vi "BLM status.vi"(2 "error in (no error)":errorcluster, 4 "Motor Address":string="0", 5 "Porty Address":refnum<visa-resource-name>) -> (0 "error out":errorcluster, 1 "Motor is moving":bool)   [LabVIEW 2019]
uses:
  BLM_IgnoreAlarms.vi
panel:
  out "BLM Status":bool[](array[boolean])
  out "Response":string
  # "SC command - Response Details:\nHex Value Status Code bit definition\n0001 Motor Enabled (Motor Disabled if this bit = 0)\n0002 Sampling (for Quick Tuner)\n0004 Drive Fault (check Alarm Code)\n0008 In Position (motor is in position)\n0010 Moving (motor is moving)\n0020 Jogging (currently in jog mode)\n0040 Stopping (in the process of stopping from a stop command)\n0080 Waiting (for an input)\n0100 Saving (parameter data is being saved)\n0200 Alarm present (check Alarm Code)\n0400 Homing (executing an SH command)\n0800 Wait Time (executing a WT command)\n1000 Wizard running (Timing Wizard is running)\n2000 Checking encoder (Timing Wizard is running)\n4000 Q Program is running\n8000 Initializing (happens at power up)"
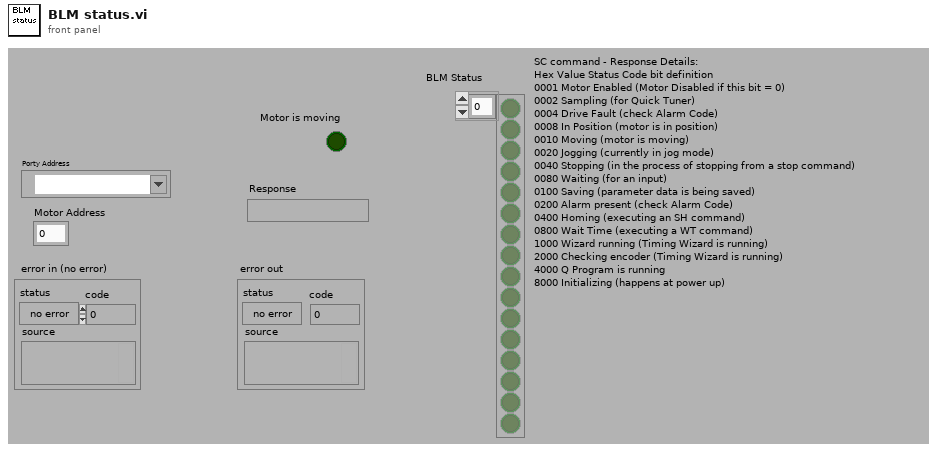
[diagram p1: front panel]
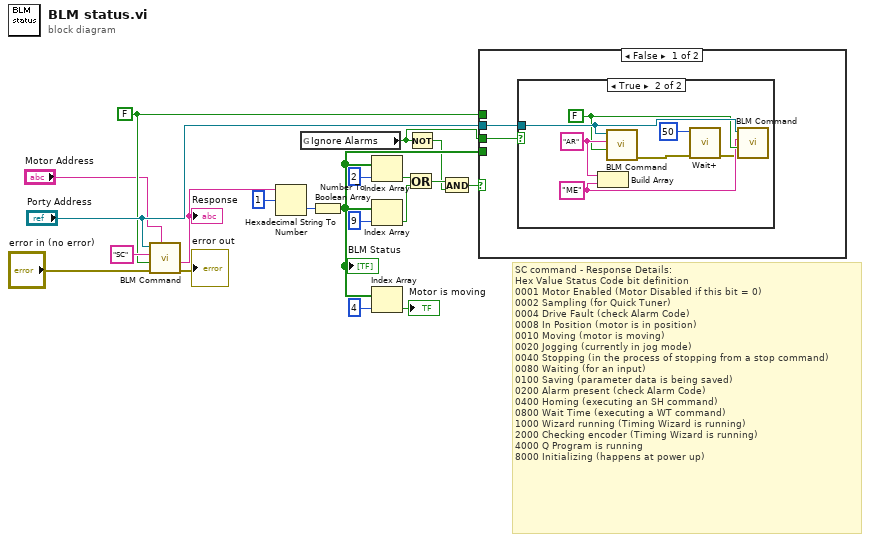
[diagram p0: block diagram]
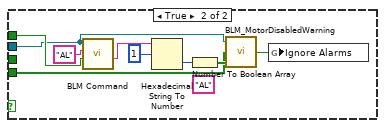
[diagram p3: hidden frame]
diagram:
  w6 = FALSE
  # "SC command - Response Details:\nHex Value Status Code bit definition\n0001 Motor Enabled (Motor Disabled if this bit = 0)\n0002 Sampling (for Quick Tuner)\n0004 Drive Fault (check Alarm Code)\n0008 In Position (motor is in position)\n0010 Moving (motor is moving)\n0020 Jogging (currently in jog mode)\n0040 Stopping (in the process of stopping from a stop command)\n0080 Waiting (for an input)\n0100 Saving (parameter data is being saved)\n0200 Alarm present (check Alarm Code)\n0400 Homing (executing an SH command)\n0800 Wait Time (executing a WT command)\n1000 Wizard running (Timing Wizard is running)\n2000 Checking encoder (Timing Wizard is running)\n4000 Q Program is running\n8000 Initializing (happens at power up)"
  n1 = call "BLM Command.vi"("Motor Address"="Motor Address", "error in (no error)"="error in (no error)", "Read Echo?"=w6, "Command"="SC", "Port Address"="Porty Address") -> ("error out"=→"error out":errorcluster, "Response"=w17:string)  [unwired: 1 in, 3 out]
  "Response" <- w17
  n2 = Hexadecimal String To Number(string=w17, offset=u32 1 ("initial scan location")) -> (number=w15:u32)  [unwired: 1 in, 1 out]
  n3 = global read "BLM_IgnoreAlarms.vi" "Ignore Alarms"() -> (w2:bool)
  n4 = Number To Boolean Array(number=w15) -> (Boolean array=w8:bool[])
  "BLM Status" <- w8
  n5 = Index Array(array=w8, index=2) -> (element=w12:bool)
  n6 = Index Array(array=w8, index=9) -> (element=w11:bool)
  n7 = Index Array(array=w8, index=4) -> (element=→"Motor is moving":bool)
  n8 = Or(x=w12, y=w11) -> (x .or. y?=w4:bool)
  n9 = Not(x=w2) -> (.not. x?=w3:bool)
  n10 = And(x=w4, y=w3) -> (x .and. y?=w5:bool)
  n11 = case shown="False" w5 {
    tunnel: w8 -> [_ w32]
    tunnel: "Porty Address" -> [w21 w31]
    tunnel: w6 -> [_ w38]
    tunnel: w2 -> [w22 _]
    frame False {
      n12 = case shown="True" w22 {
        tunnel: w21 -> [_ w28]
        frame False {
        }
        frame True {
          w26 = "ME" ("Command")
          w27 = FALSE ("Read Echo?")
          w29 = "AR" ("Command")
          n13 = Build Array(w29, w26) -> ()  [unwired: 1 out]
          n14 = call "BLM Command.vi"("Read Echo?"=w27, "Command"=w29, "Port Address"=w28) -> ("error out"=w25:errorcluster)  [unwired: 3 in, 4 out]
          n15 = call "Wait+.vi"("Error In"=w25, "milliseconds to wait"=u32 50) -> ("Error Out"=w24:errorcluster)  [unwired: 4 in, 1 out]
          n16 = call "BLM Command.vi"("error in (no error)"=w24, "Read Echo?"=w27, "Command"=w26, "Port Address"=w28) -> ()  [unwired: 2 in, 5 out]
        }
      }
    }
    frame True {
      (unwired) "AL" ("Command")
      n17 = call "BLM Command.vi"("Read Echo?"=w38, "Command"="AL", "Port Address"=w31) -> ("Response"=w34:string)  [unwired: 3 in, 4 out]
      n18 = Hexadecimal String To Number(string=w34, offset=u32 1 ("initial scan location")) -> (number=w36:u32)  [unwired: 1 in, 1 out]
      n19 = Number To Boolean Array(number=w36) -> (Boolean array=w33:bool[])
      n20 = call "BLM_MotorDisabledWarning.vi"("BLM Alarm Code"=w33, "BLM Status"=w32, "Instrument Address"=w31) -> ("Ignore Alarms"=w30:bool)  [unwired: 1 in, 1 out]
      n21 = global write "BLM_IgnoreAlarms.vi" "Ignore Alarms"(w30) -> ()
    }
  }
